vi "Retrieve Outputs.vi"(7 "SMO in":refnum<class "SMO.lvclass">, 8 "error in (no error)":errorcluster, 11 "API":T1) -> (0 "error out":errorcluster, 2 "Output":variant, 3 "API dup":T1, 5 "SMO out":refnum<class "SMO.lvclass">)   [LabVIEW 2021, in "smo.lvlib" / "SMOFacade.lvclass"]
uses:
  SMOFacade.lvclass
  SMO/SMO.lvclass
  Registry/SMO_API--Cluster.ctl
  Terminal/Terminal.lvclass
  SMOFacade.lvclass/SMOFacade.ctl
  smo.lvlib
  Registry/Registry-SMO.lvclass
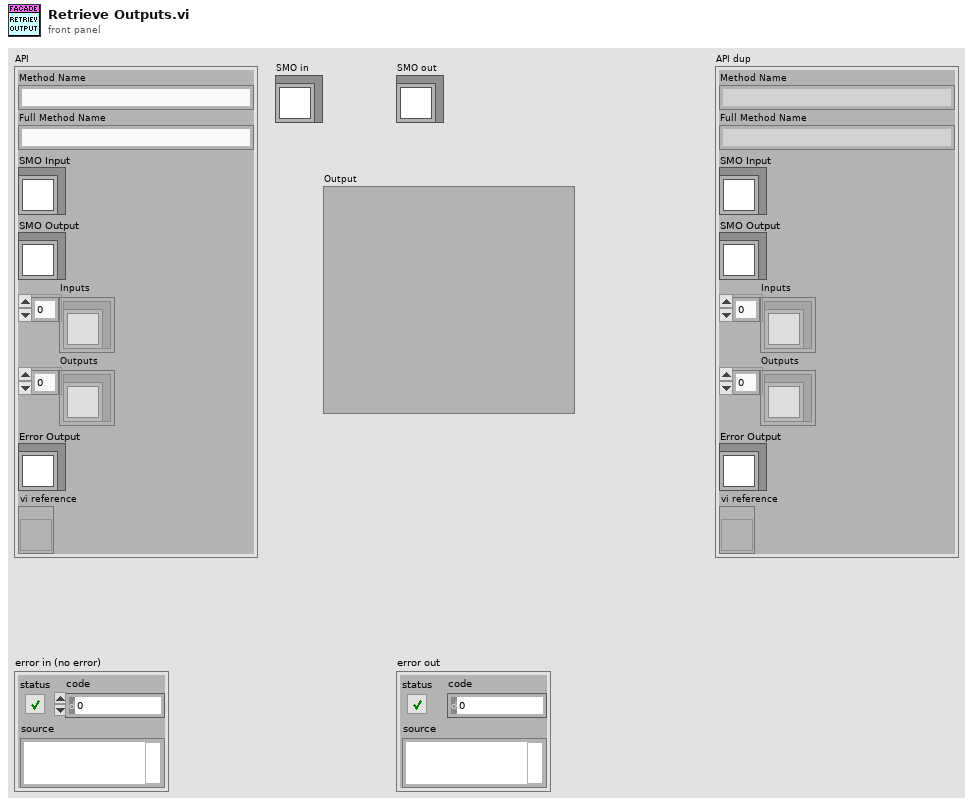
[diagram p1: front panel]
types:
  T1 = typedef "smo.lvlib/Registry-SMO.lvclass/SMO_API--Cluster.ctl" = cluster{"Method Name":string, "Full Method Name":string, "SMO Input":refnum<class "Terminal.lvclass">, "SMO Output":refnum<class "Terminal.lvclass">, "Inputs":refnum<class "Terminal.lvclass">[], "Outputs":refnum<class "Terminal.lvclass">[], "Error Output":refnum<class "Terminal.lvclass">, "vi reference":refnum<vi>}
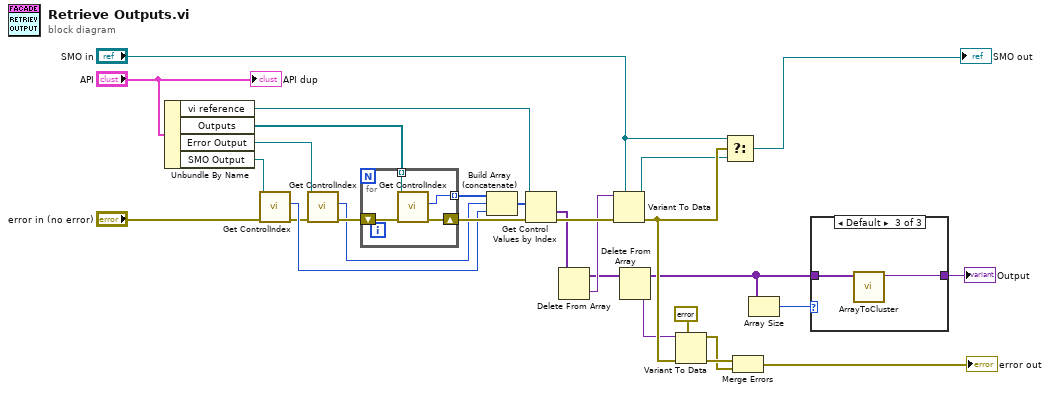
[diagram p0: block diagram]
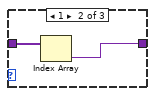
[diagram p3: hidden frame]
diagram:
  n1 = Unbundle By Name("API") -> ("vi reference"=w12:refnum<vi>, "Outputs"=w20:refnum<class "Terminal.lvclass">[], "Error Output"=w11:refnum<class "Terminal.lvclass">, "SMO Output"=w16:refnum<class "Terminal.lvclass">)
  n2 = call "Get ControlIndex.vi"("error in (no error)"="error in (no error)", "Terminal in"=w16) -> ("error out"=w14:errorcluster, "ControlIndex"=w15:i32)  [unwired: 7 in, 1 out]
  n3 = call "Get ControlIndex.vi"("error in (no error)"=w14, "Terminal in"=w11) -> ("error out"=w18:errorcluster, "ControlIndex"=w17:i32)  [unwired: 7 in, 1 out]
  n4 = for {
    tunnel: [w33] -> w5 mode=indexing
    shift-right: [w31] -> w19
    shift-left: w18 -> [w32]
    tunnel: w20 -> [w30] mode=indexing
    n5 = call "Get ControlIndex.vi"("error in (no error)"=w32, "Terminal in"=w30) -> ("error out"=w31:errorcluster, "ControlIndex"=w33:i32)  [unwired: 7 in, 1 out]
  }
  n6 = Build Array (concatenate)(w5, w17, w15) -> (w4:i32[])
  n7 = Get Control Values by Index(0:w12, 1:w4, 3:w19) -> (10:w6:variant[], 11:w24:errorcluster)
  n8 = Delete From Array(array=w6) -> (deleted portion=w21:variant, array with subset deleted=w8:variant[])  [unwired: 2 in]
  n9 = Variant To Data(error in=w24, type="SMO in", Variant=w21) -> (data=w26:refnum<class "SMO.lvclass">, error out=w29:errorcluster)
  n10 = Delete From Array(array=w8) -> (deleted portion=w10:variant, array with subset deleted=w9:variant[])  [unwired: 2 in]
  n11 = Variant To Data(error in=w29, type=errorcluster {"status"=FALSE, "code"=0, "source"=""} ("error out"), Variant=w10) -> (data=w7:errorcluster, error out=w23:errorcluster)
  n12 = Select(t="SMO in", s=w29, f=w26) -> (s? t:f=→"SMO out":refnum<class "SMO.lvclass">)
  n13 = Merge Errors(w23, w7) -> (→"error out":errorcluster)
  n14 = Array Size(array=w9) -> (size(s)=w2:i32)
  n15 = case shown="Default" w2 {
    tunnel: w9 -> [_ w35 w37]
    tunnel: [_ w34 w36] -> w3
    frame 0 {
    }
    frame 1 {
      n16 = Index Array(array=w35) -> (element=w34:variant)  [unwired: 1 in]
    }
    frame Default {
      n17 = call "ArrayToCluster.vi"("Array"=w37) -> ("Cluster"=w36:variant)  [unwired: 10 in]
    }
  }
  "Output" <- w3
  "API dup" <- "API"
